vi "data_logger_comparator.vi"() -> ()   [LabVIEW 2015]
panel:
  in  "Array":path[](array[path])
  out "x .or. y?":bool
  in  "milliseconds to wait":u32
  out "error out 2":errorcluster
  out "error out 1":errorcluster
  out "String 1":string
  out "s? t:f":bool
  out "default (0 I32) 2":i32
  out "default (0 I32)":i32
  in  "Path 2":path
  in  "Path":path
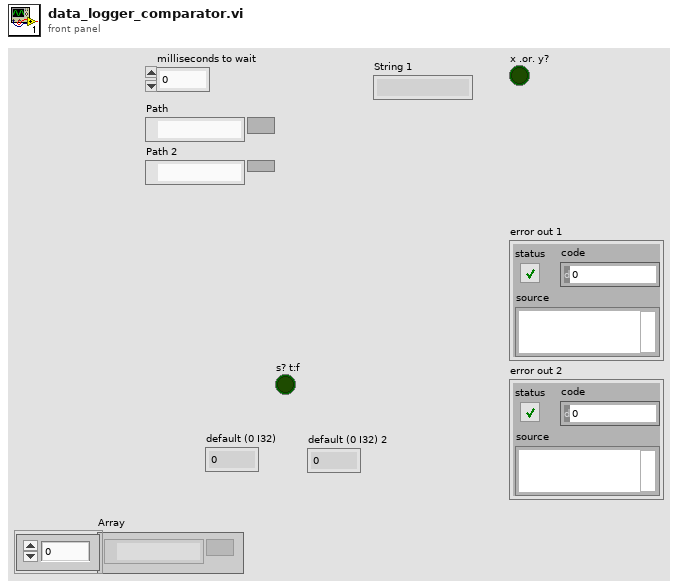
[diagram p1: front panel]
types:
  T1 = enum16{"open", "replace", "create", "open or create", "replace or create", "replace or create with confirmation"}
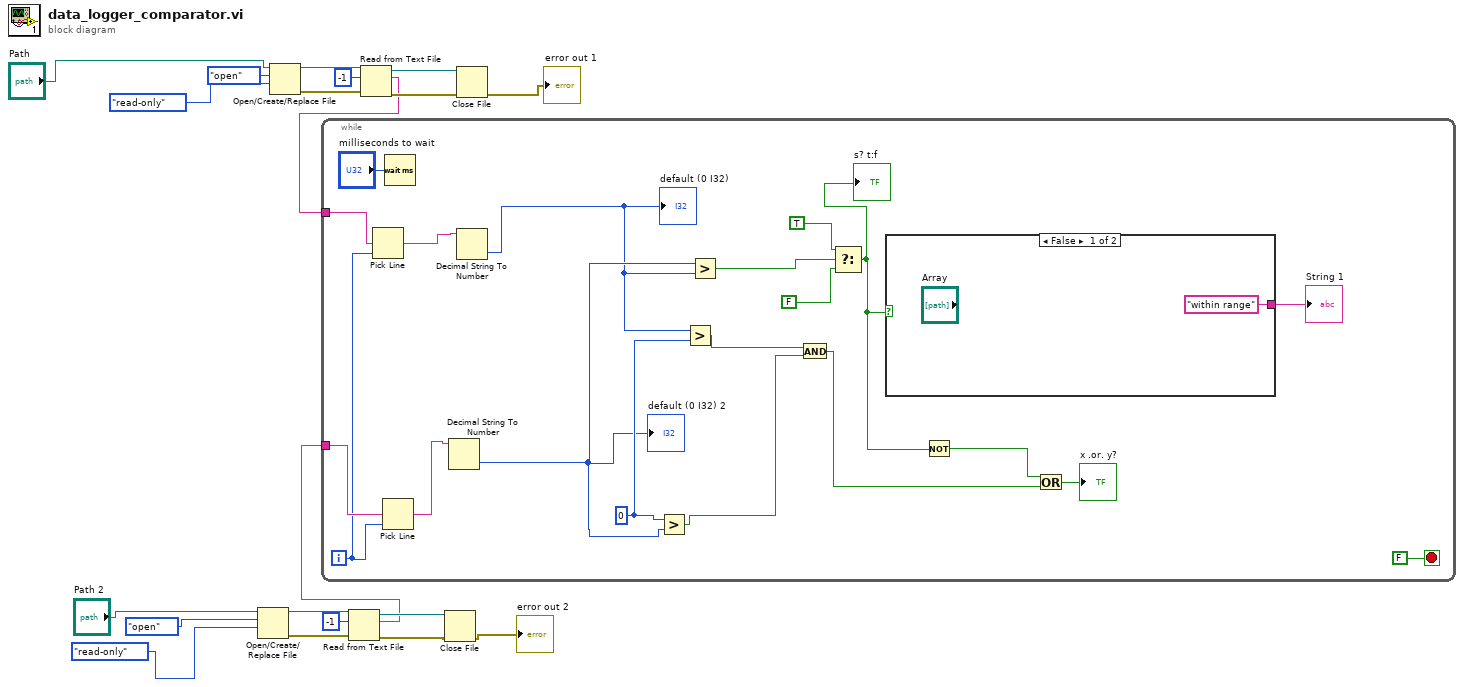
[diagram p0: block diagram]
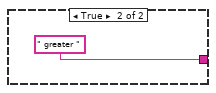
[diagram p2: hidden frame]
diagram:
  n1 = Open/Create/Replace File(file path (use dialog)="Path 2", operation (0:open)=T1."open", access (0:read/write)=enum16{"read/write", "read-only", "write-only"}."read-only") -> (refnum out=w14:refnum<file>, error out=w13:errorcluster)  [unwired: 3 in, 1 out]
  n2 = Open/Create/Replace File(file path (use dialog)="Path", operation (0:open)=T1."open", access (0:read/write)=enum16{"read/write", "read-only", "write-only"}."read-only") -> (refnum out=w20:refnum<file>, error out=w19:errorcluster)  [unwired: 3 in, 1 out]
  n3 = Read from Text File(file (use dialog)=w14, count=-1, error in=w13) -> (refnum out=w7:refnum<file>, text=w1:string, error out=w8:errorcluster)  [unwired: 1 in, 1 out]
  n4 = Read from Text File(file (use dialog)=w20, count=-1, error in=w19) -> (refnum out=w17:refnum<file>, text=w15:string, error out=w16:errorcluster)  [unwired: 1 in, 1 out]
  n5 = while {
    tunnel: w15 -> [w28]
    tunnel: w1 -> [w30]
    i -> [w24]
    stop <- FALSE stop-if-true
    w35 = 0 ("x")
    n6 = Pick Line(multi-line string=w28, line index=w24) -> (output string=w27:string)  [unwired: 1 in]
    n7 = Pick Line(multi-line string=w30, line index=w24) -> (output string=w29:string)  [unwired: 1 in]
    n8 = Wait (ms)(milliseconds to wait="milliseconds to wait") -> ()  [unwired: 1 out]
    n9 = Decimal String To Number(string=w29) -> (number=w31:i32)  [unwired: 2 in, 1 out]
    "default (0 I32) 2" <- w31
    n10 = Decimal String To Number(string=w27) -> (number=w25:i32)  [unwired: 2 in, 1 out]
    "default (0 I32)" <- w25
    n11 = Greater?(x=w35, y=w31) -> (0:w37:bool)
    n12 = Greater?(x=w25, y=w35) -> (0:w36:bool)
    n13 = Greater?(x=w31, y=w25) -> (0:w40:bool)
    n14 = And(x=w36, y=w37) -> (x .and. y?=w34:bool)
    n15 = Select(t=TRUE, s=w40, f=FALSE) -> (s? t:f=w32:bool)
    "s? t:f" <- w32
    n16 = case shown="False" w32 {
      tunnel: ["within range" " greater "] -> w26
      frame False {
      }
      frame True {
      }
    }
    "String 1" <- w26
    n17 = Not(x=w32) -> (.not. x?=w33:bool)
    n18 = Or(x=w33, y=w34) -> (x .or. y?=→"x .or. y?":bool)
  }
  n19 = Close File(refnum=w7, error in=w8) -> (error out=→"error out 2":errorcluster)  [unwired: 1 out]
  n20 = Close File(refnum=w17, error in=w16) -> (error out=→"error out 1":errorcluster)  [unwired: 1 out]
